vi "Set Active Scale.vi"(8 "error in (no error)":errorcluster, 10 "references":T1, 11 "Index":i32) -> (0 "error out":errorcluster)   [LabVIEW 2013, in "Scaling editor node.lvclass"]
uses:
  Scaling editor node.lvclass
  <vilib>/NI/DCAF/Tag Editor Core/Table API/Table Manager/object ref.ctl
  <vilib>/NI/DCAF/Tag Editor Core/Configuration Editor/Classes/Engine Parent/Engine Parent Editor Node.lvclass
  <vilib>/NI/DCAF/Tag Editor Core/Configuration Editor/Classes/Module editor node/module editor node.lvclass
  Scaling editor node.lvclass/Scaling editor node.ctl
  accessors/Write active scale index .vi
  <vilib>/NI/DCAF/Tag Editor Core/Table API/Table Manager/Table Manager.lvclass
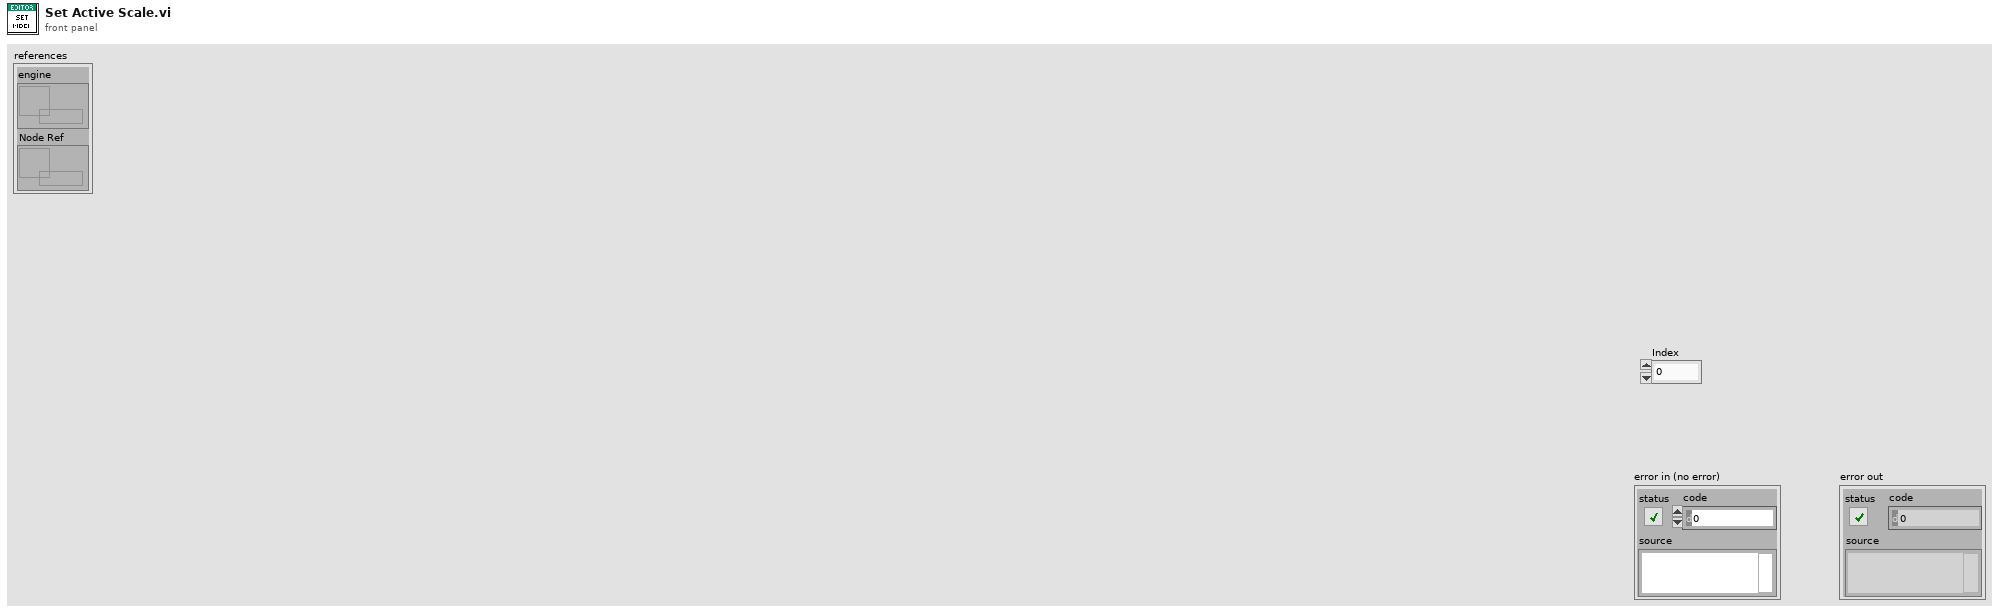
[diagram p1: front panel]
types:
  T1 = typedef "Table Manager.lvlib/Table Manager.lvclass/object ref.ctl" = cluster{"engine":refnum<data-value>, "Node Ref":refnum<data-value>}
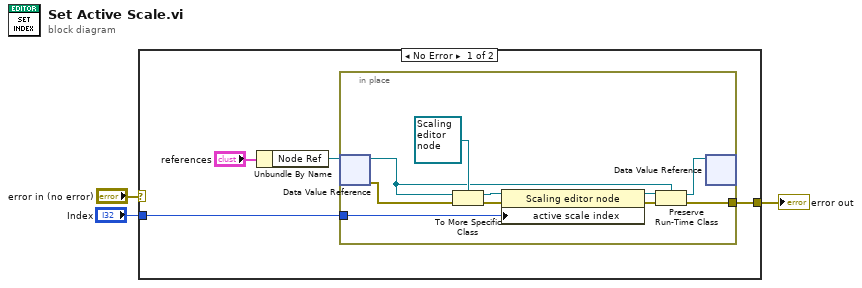
[diagram p0: block diagram]
diagram:
  n1 = case shown="No Error" "error in (no error)" {
    selector: "error in (no error)" -> [_ w18]
    tunnel: [w7 w18] -> w1
    tunnel: "Index" -> [w4 _]
    frame No Error {
      n2 = Unbundle By Name("references") -> ("Node Ref"=w5:refnum<data-value>)
      n3 = in-place {
        in-place-border: [w11] -> w7
        in-place-border: w4 -> [w15]
        n4 = in-place-dvr #1(w5) -> (w9:refnum<class "module editor node.lvclass">, w14:errorcluster)
        n5 = To More Specific Class(target class=refnum<class "Scaling editor node.lvclass"> refnum ("Scaling editor node"), reference=w9, error in=w14) -> (specific class reference=w17:refnum<class "Scaling editor node.lvclass">, error out=w16:errorcluster)
        n6 = property class="Scaling editor node"(reference=w17, error in=w16, "active scale index "=w15) -> (reference out=w10:refnum<class "Scaling editor node.lvclass">, error out=w12:errorcluster)
        n7 = Preserve Run-Time Class(object in=w10, error in=w12, 2:w9) -> (object out=w8:refnum<class "module editor node.lvclass">, error out=w11:errorcluster)
        n8 = in-place-dvr #1(w8) -> ()  [unwired: 2 out]
      }
    }
    frame Error {
    }
  }
  "error out" <- w1
